vi "Eval Polar to Rect.vi"(4 "radius as function of angle":string, 5 "end":dbl=1.0 format="%.2f", 6 "start":dbl format="%.2f", 7 "number of points":u32=10) -> (0 "error":i32, 1 "ticks":u32, 2 "Y":dbl[](array[numeric]) format="%.2f", 3 "X":dbl[](array[numeric]) format="%.2f")   [LabVIEW 2017, in "NI_Gmath.lvlib"]
doc: "Calculates the values of a polar parametric curve in 2D."
uses:
  <vilib>/gmath/NI_Gmath.lvlib
panel:
  # "Example:\n\n number of points: 100 \n start: 0.0\n end: 1.0\n radius as function of angle: t*t+exp(-t)"
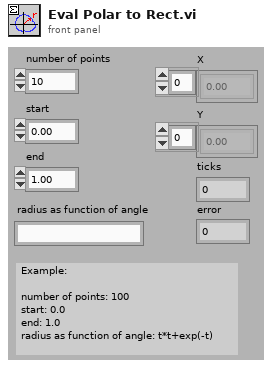
[diagram p1: front panel]
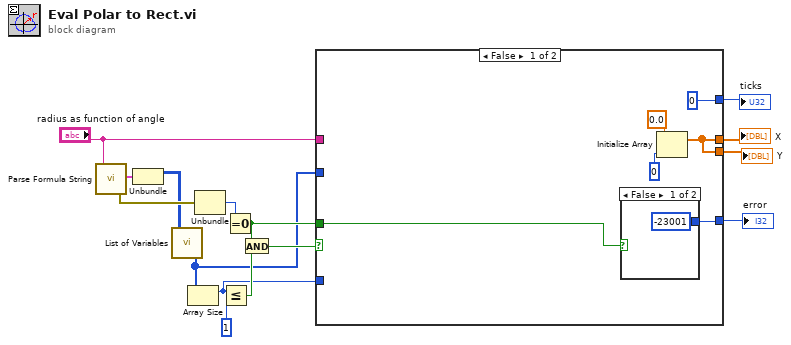
[diagram p0: block diagram]
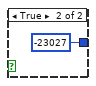
[diagram p2: hidden frame]
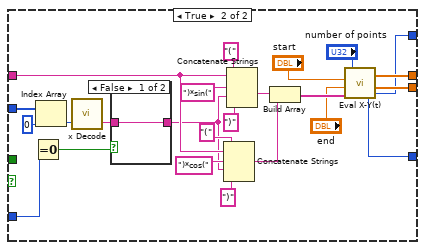
[diagram p3: hidden frame]
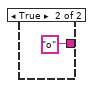
[diagram p4: hidden frame]
diagram:
  n1 = call <vilib>:"Parse Formula String.vi"("formula"="radius as function of angle") -> ("error out"=w10:errorcluster, "Parsed Formula"=w2:cluster{"Table":i32[][], "Y Values":dbl[]})  [unwired: 1 in]
  n2 = Unbundle(w2) -> ("Table"=w1:i32[][])  [unwired: 1 out]
  n3 = call <vilib>:"List of Variables.vi"("Table"=w1) -> ("List of variables"=w5:i32[])
  n4 = Array Size(array=w5) -> (size(s)=w3:i32)
  n5 = Unbundle(w10) -> ("code"=w6:i32)  [unwired: 2 out]
  n6 = Less Or Equal?(x=w3, y=1) -> (x <= y?=w9:bool)
  n7 = Equal To 0?(x=w6) -> (x = 0?=w12:bool)
  n8 = And(x=w12, y=w9) -> (x .and. y?=w8:bool)
  n9 = case shown="False" w8 {
    tunnel: "radius as function of angle" -> [_ w47]
    tunnel: [w17 w46] -> w14
    tunnel: [w17 w45] -> w15
    tunnel: [w18 w34] -> w7
    tunnel: w12 -> [w19 _]
    tunnel: w5 -> [_ w32]
    tunnel: [u32 0 w30] -> w4
    tunnel: w3 -> [_ w27]
    frame False {
      n10 = case shown="False" w19 {
        tunnel: [-23001 -23027] -> w18
        frame False {
        }
        frame True {
        }
      }
      n11 = Initialize Array(0.0, 0) -> (w17:dbl[])
    }
    frame True {
      n12 = Equal To 0?(x=w27) -> (x = 0?=w26:bool)
      n13 = Index Array(array=w32, index=0) -> (element=w31:i32)
      n14 = call <vilib>:"x Decode.vi"("number"=w31) -> ("x string"=w25:string)  [unwired: 1 in, 1 out]
      n15 = case shown="False" w26 {
        tunnel: w25 -> [w48 _]
        tunnel: [w48 "o"] -> w24
        frame False {
        }
        frame True {
        }
      }
      n16 = Concatenate Strings("(", w47, ")*cos(", w24, ")") -> (w41:string)
      n17 = Concatenate Strings("(", w47, ")*sin(", w24, ")") -> (w40:string)
      n18 = Build Array(w40, w41) -> (w44:string[])
      n19 = call <vilib>:"Eval X-Y(t).vi"("Formulas"=w44, "end"="end", "start"="start", "number of points"="number of points") -> ("error"=w34:i32, "ticks"=w30:u32, "Y"=w46:dbl[], "X"=w45:dbl[])
    }
  }
  "X" <- w15
  "Y" <- w14
  "error" <- w7
  "ticks" <- w4
